vi "Read System Ring Refnum.vi"(8 "error in (no error)":errorcluster, 11 "Manager in":refnum<class "Manager.lvclass">) -> (0 "error out":errorcluster, 2 "System Ring Refnum":refnum<vi>, 3 "Manager out":refnum<class "Manager.lvclass">)   [LabVIEW 2013, in "Manager.lvlib" / "Manager.lvclass"]
uses:
  Manager.lvclass
  Manager.lvclass/Manager.ctl
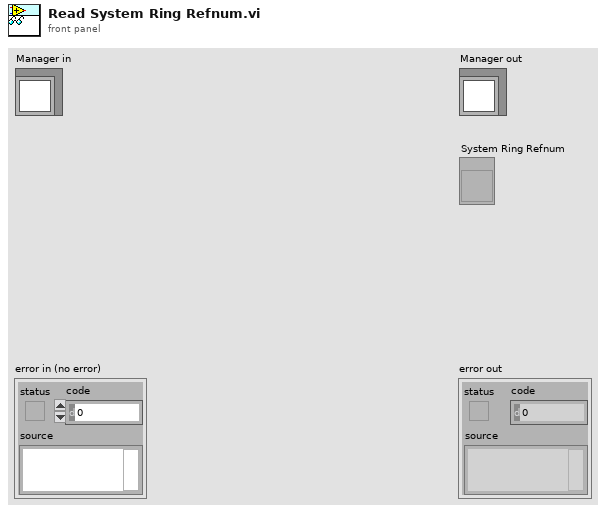
[diagram p1: front panel]
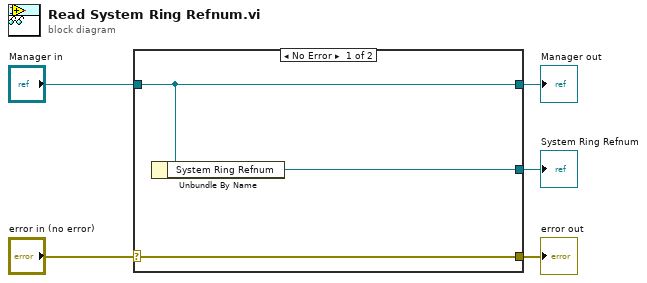
[diagram p0: block diagram]
diagram:
  n1 = case shown="No Error" "error in (no error)" {
    selector: "error in (no error)" -> [w8 w9]
    tunnel: [w8 w9] -> w4
    tunnel: [w7 w10] -> w2
    tunnel: "Manager in" -> [w7 w10]
    tunnel: [w6 _] -> w1
    frame No Error {
      n2 = Unbundle By Name(w7) -> ("System Ring Refnum"=w6:refnum<vi>)
    }
    frame Error {
    }
  }
  "error out" <- w4
  "Manager out" <- w2
  "System Ring Refnum" <- w1
